vi "BaxterInit.vi"   [LabVIEW 2012]
doc: "Enables motors, calibrates grippers"
uses:
  <userlib>/rosforlv/ROS/Code/SubVIs/BaxterSide.ctl
types:
  T1 = typedef "BaxterSide.ctl" = enum16{"left", "right"}
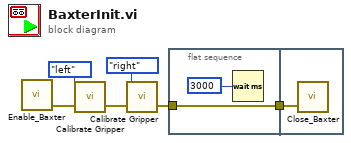
[diagram p0: block diagram]
diagram:
  n1 = call <userlib>:"Enable_Baxter.vi"() -> ("error out"=w6:errorcluster)  [unwired: 4 in]
  n2 = call <userlib>:"Calibrate Gripper.vi"("Side"=BaxterSide."left", "error in"=w6) -> ("error out"=w4:errorcluster)  [unwired: 4 in]
  n3 = call <userlib>:"Calibrate Gripper.vi"("Side"=BaxterSide."right", "error in"=w4) -> ("error out"=w2:errorcluster)  [unwired: 4 in]
  n4 = flat-sequence {
    tunnel: w2 -> [w8]
    tunnel: [w8] -> w3
    tunnel: w3 -> [w9]
    frame #0 {
      n5 = Wait (ms)(milliseconds to wait=u32 3000) -> ()  [unwired: 1 out]
    }
    frame #1 {
      n6 = call <userlib>:"Close_Baxter.vi"("error in"=w9) -> ()  [unwired: 3 in, 1 out]
    }
  }
